vi "SHOOT.vi"(10 "argv":string[](array[string]), 11 "args":u8) -> ()   [LabVIEW 2014]
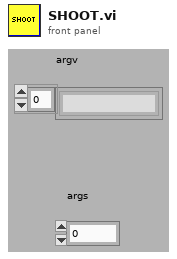
[diagram p1: front panel]
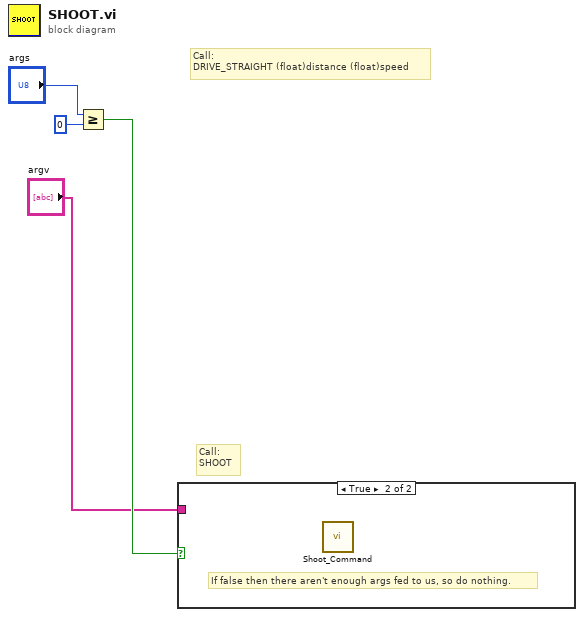
[diagram p0: block diagram]
diagram:
  # "Call:\nSHOOT"
  # "Call:\nDRIVE_STRAIGHT (float)distance (float)speed"
  n1 = Greater Or Equal?(x="args", y=u8 0) -> (x >= y?=w4:bool)
  n2 = case shown="True" w4 {
    tunnel: "argv" -> [_ _]
    frame False {
    }
    frame True {
      # "If false then there aren't enough args fed to us, so do nothing."
      n3 = call "Shoot_Command.vi"() -> ()  [unwired: 12 in]
    }
  }
